vi "Retriggerable_Finite_Counter_20230323_v2019.vi"() -> ()   [LabVIEW 2019]
uses:
  <resource>/objmgr/daqmx.rc
  <vilib>/Utility/error.llb/DialogType.ctl
  <vilib>/DAQmx/configure/timing.llb/DAQmx Timing (Sample Clock).vi
  <vilib>/DAQmx/create/channels.llb/DAQmx Create Channel (CI-Count Edges).vi
  <vilib>/DAQmx/read.llb/DAQmx Read (Counter 1D U32 1Chan NSamp).vi
  <vilib>/DAQmx/create/channels.llb/DAQmx Create Channel (AI-Voltage-Basic).vi
  <vilib>/DAQmx/configure/timing.llb/DAQmx Timing (Implicit).vi
  <vilib>/DAQmx/create/channels.llb/DAQmx Create Channel (CO-Pulse Generation-Frequency).vi
  <vilib>/DAQmx/read.llb/DAQmx Read (Analog 1D Wfm NChan NSamp).vi
  <vilib>/DAQmx/configure/events/hardwareSignals.llb/DAQmx Export Signal (Most Signals).vi
panel:
  in  "AI Physical Channel":tag="Dev2/ai0"
  out "Read Iteration.":i32=20 caption="Read Iteration.\nIf working correctly,\nthis should increment\nonce per second."
  out "Actual Duty Cycle":dbl=0.01
  out "Actual Frequency":dbl=1.0
  in  "Duty Cycle":dbl=0.01 caption="Duty Cycle Must Be Less Than Sampling Duration (%)" format="%.6f"
  in  "Frequency (Hz)":dbl=1.0 format="%.6f"
  in  "Output Terminal":tag="/Dev2/PFI12" caption="Output Terminal For Routing to First Counter"
  in  "Counter 2":tag="Dev2/ctr1"
  out "Total Count\nThis is the":u32 caption="Total Count.\nThis is what you're most interested in."
  in  "Stop":bool
  in  "Trigger Type":enum32{"No Trigger", "Digital Arm Start"}(tab)=enum."Digital Arm Start"
  in  "Edge":i32(ring)=10280 items=["Rising"=10280, "Falling"=10171]
  out "Data":u32[](array[numeric])
  in  "Samples":i32=1000
  in  "Signal Input Terminal":tag="PFI8"
  in  "Counter":tag="Dev2/ctr0"
  in  "Sample Rate":dbl=100000.0
  in  "Sample Clock Source":tag="/Dev2/PFI14"
  # "Task 1: Finite Counter Measurement"
  # "Task 2: Create Sample Clock"
  # "Task 2: Create Slow Pulse Train"
  # "Lots of count values. (You can delete this indicator.\nI've left it here to make it easier to understand how this is working.)"
  # "To configure and use a trigger or the count reset you must have the \"Digital Arm Start\"  tab selected."
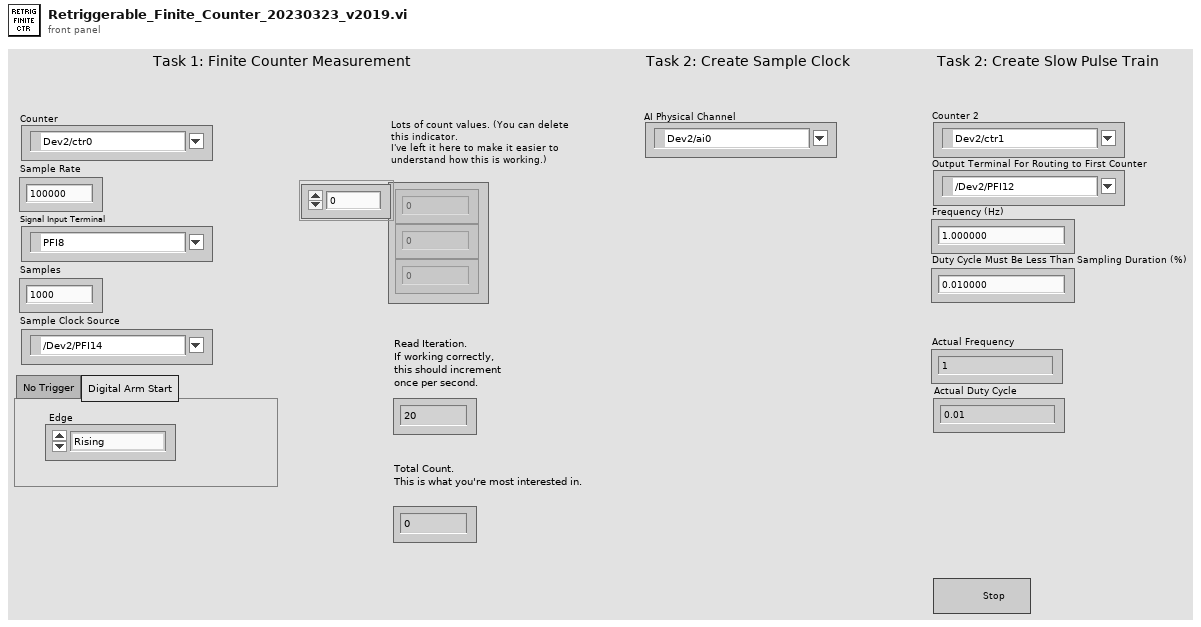
[diagram p1: front panel]
types:
  T1 = typedef "DialogType.ctl" = u16
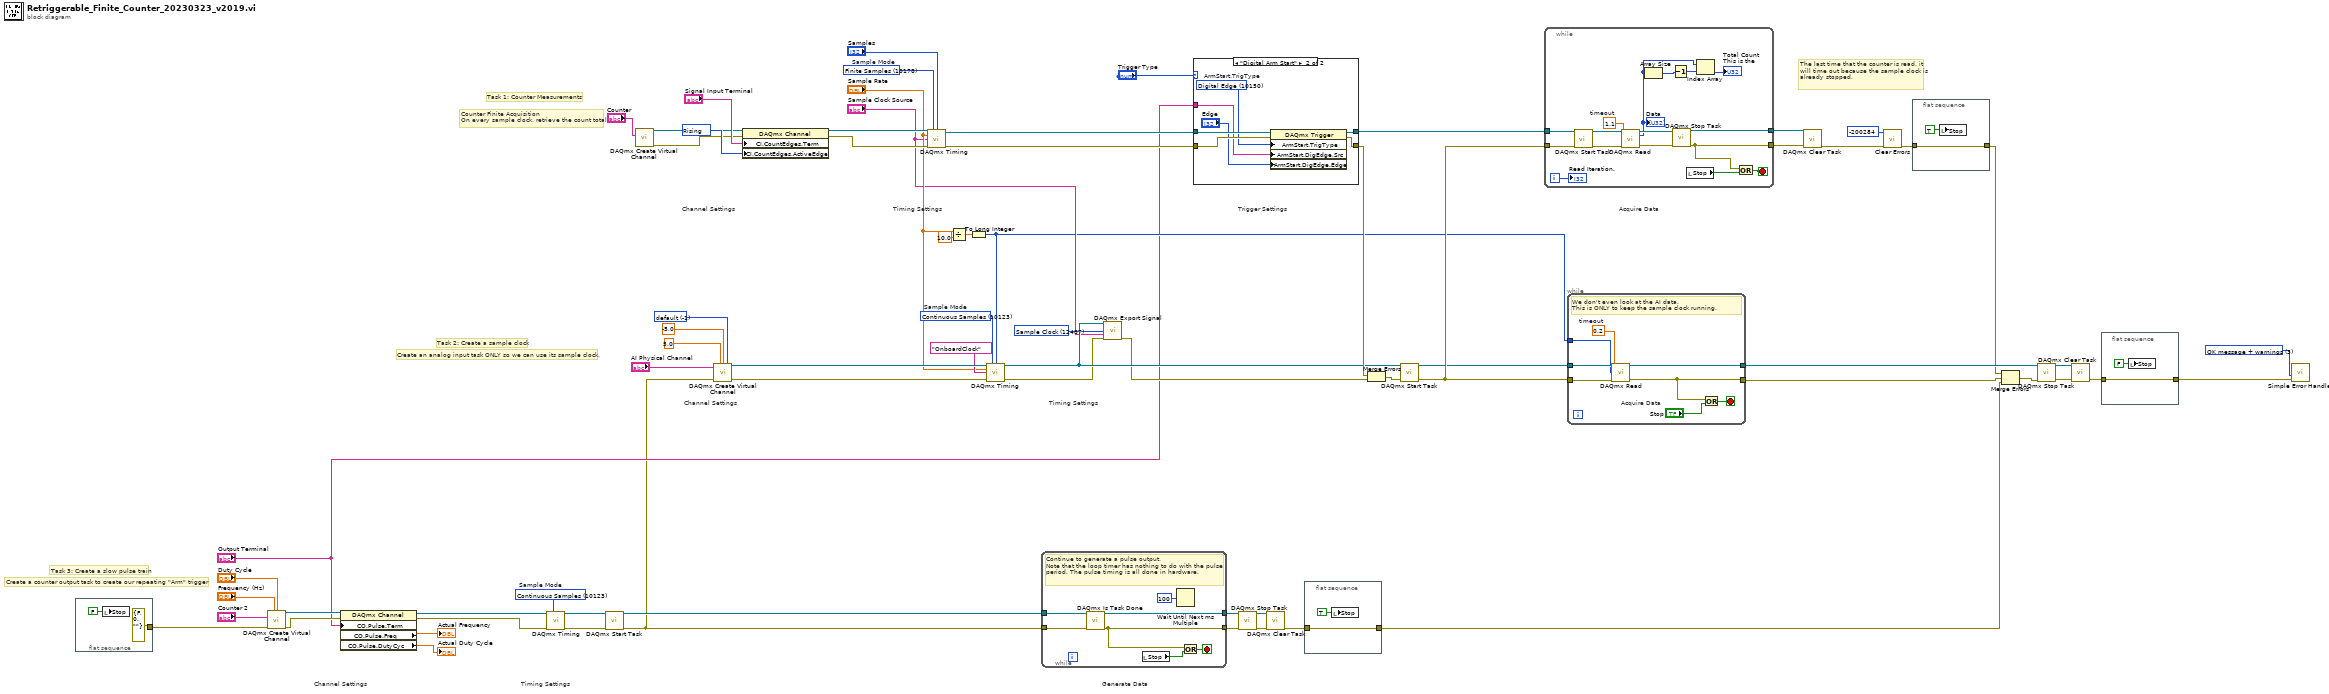
[diagram p0: block diagram]
diagram:
  w69 = 10280 items=["Rising"=10280, "Falling"=10171] ("Active Edge")
  w27 = 10123 items=["Finite Samples"=10178, "Continuous Samples"=10123, "Hardware Timed Single Point"=12522]  # Sample Mode
  w33 = 12487 items=["AI Convert Clock"=12484, "10MHz Reference Clock"=12536, "20MHz Timebase Clock"=12486, "Sample Clock"=12487, "Advance Trigger"=12488, "Reference Trigger"=12490, "Start Trigger"=12491, "Advance Complete Event"=12492, "AI Hold Complete Event"=12493, "Counter Output Event"=12494, "Change Detection Event"=12511, "Watchdog Timer Expired Event"=12512] ("signal")
  w53 = -1 items=["default"=-1, "RSE"=10083, "NRSE"=10078, "Differential"=10106, "Pseudodifferential"=12529] ("Terminal Configuration")
  w46 = T1 3 items=["no dialog", "OK message", "continue or stop message", "OK message + warnings", "continue/stop + warnings"] ("type of dialog (OK msg:1)")
  w57 = 10123 items=["Finite Samples"=10178, "Continuous Samples"=10123, "Hardware Timed Single Point"=12522]  # Sample Mode
  w68 = 10178 items=["Finite Samples"=10178, "Continuous Samples"=10123, "Hardware Timed Single Point"=12522]  # Sample Mode
  # "Task 3: Create a slow pulse train"
  # "Task 2: Create a sample clock"
  # "Task 1: Counter Measurements"
  # "The last time that the counter is read, it will time out because the sample clock is already stopped."
  # "Create a counter output task to create our repeating \"Arm\" trigger"
  # "Generate Data"
  # "Timing Settings"
  # "Channel Settings"
  # "Create an analog input task ONLY so we can use its sample clock."
  # "Counter Finite Acquisition\nOn every sample clock, retrieve the count total"
  # "Acquire Data"
  # "Timing Settings"
  # "Channel Settings"
  # "Acquire Data"
  # "Trigger Settings"
  # "Timing Settings"
  # "Channel Settings"
  n1 = flat-sequence {
    tunnel: [errorcluster {"status"=FALSE, "code"=0, "source"=""} ("error out")] -> w6
    frame #0 {
      n2 = local write "Stop"(FALSE ("Stop")) -> ()
    }
  }
  n3 = call-poly <vilib>:"DAQmx Create Virtual Channel.vi"("frequency"="Frequency (Hz)", "duty cycle"="Duty Cycle", "counter"="Counter 2", "error in"=w6) -> ("task out"=w22:refnum<k21>, "error out"=w21:errorcluster)  [unwired: 10 in]
  n4 = property class="DAQmx Channel"(reference=w22, error in=w21, "CO.Pulse.Term"="Output Terminal") -> (reference out=w19:refnum<k21>, error out=w20:errorcluster, "CO.Pulse.Freq"=→"Actual Frequency":dbl, "CO.Pulse.DutyCyc"=→"Actual Duty Cycle":dbl)
  n5 = call-poly <vilib>:"DAQmx Timing.vi"("task/channels in"=w19, "sample mode"=w27, "error in"=w20) -> ("task out"=w24:refnum<k21>, "error out"=w23:errorcluster)  [unwired: 11 in]
  n6 = call <vilib>:"DAQmx Start Task.vi"("task/channels in"=w24, "error in"=w23) -> ("task out"=w26:refnum<k21>, "error out"=w7:errorcluster)  [unwired: 12 in]
  n7 = call-poly <vilib>:"DAQmx Create Virtual Channel.vi"("counter"="Counter") -> ("task out"=w66:refnum<k21>, "error out"=w63:errorcluster)  [unwired: 13 in]
  n8 = call-poly <vilib>:"DAQmx Create Virtual Channel.vi"("maximum value"=5.0 ("Max Voltage"), "minimum value"=-5.0 ("Min Voltage"), "input terminal configuration"=w53, "physical channels"="AI Physical Channel", "error in"=w7) -> ("task out"=w55:refnum<k21>, "error out"=w56:errorcluster)  [unwired: 9 in]
  n9 = property class="DAQmx Channel"(reference=w66, error in=w63, "CI.CountEdges.Term"="Signal Input Terminal", "CI.CountEdges.ActiveEdge"=w69) -> (reference out=w65:refnum<k21>, error out=w64:errorcluster)
  n10 = call-poly <vilib>:"DAQmx Timing.vi"("task/channels in"=w65, "sample mode"=w68, "samples per channel"="Samples", "rate"="Sample Rate", "source"="Sample Clock Source", "error in"=w64) -> ("task out"=w59:refnum<k21>, "error out"=w60:errorcluster)  [unwired: 8 in]
  n11 = Divide(x="Sample Rate", y=10.0) -> (x/y=w37:dbl)
  n12 = To Long Integer(number=w37) -> (32bit integer=w30:i32)
  n13 = call-poly <vilib>:"DAQmx Timing.vi"("task/channels in"=w55, "sample mode"=w57, "samples per channel"=w30, "rate"="Sample Rate", "source"=tag "OnboardClock" ("Sample Clock Source 2"), "error in"=w56) -> ("task out"=w36:refnum<k21>, "error out"=w35:errorcluster)  [unwired: 8 in]
  n14 = while {
    tunnel: w26 -> [w79]
    tunnel: w7 -> [w78]
    tunnel: [w75] -> w11
    tunnel: [w76] -> w12
    stop <- w77 stop-if-true
    # "Continue to generate a pulse output. \nNote that the loop timer has nothing to do with the pulse period. The pulse timing is all done in hardware."
    n15 = call <vilib>:"DAQmx Is Task Done.vi"("task/channels in"=w79, "error in"=w78) -> ("task out"=w76:refnum<k21>, "error out"=w75:errorcluster)  [unwired: 11 in, 1 out]
    n16 = local read "Stop"() -> (w73:bool)
    n17 = Wait Until Next ms Multiple(millisecond multiple=u32 100) -> ()  [unwired: 1 out]
    n18 = Or(x=w75, y=w73) -> (x .or. y?=w77:bool)
  }
  n19 = call-poly <vilib>:"DAQmx Export Signal.vi"("task/channels in"=w36, "signal"=w33, "output terminal"="Sample Clock Source", "error in"=w35) -> ("error out"=w34:errorcluster)  [unwired: 10 in, 1 out]
  n20 = case shown="\"Digital Arm Start\"" "Trigger Type" {
    tunnel: w59 -> [w81 w88]
    tunnel: w60 -> [w80 w85]
    tunnel: [w81 w87] -> w58
    tunnel: [w80 w86] -> w44
    tunnel: "Output Terminal" -> [_ w82]
    frame "No Trigger", Default {
    }
    frame "Digital Arm Start" {
      w83 = 10150 items=["Digital Edge"=10150, "None"=10230]  # ArmStart.TrigType
      n21 = property class="DAQmx Trigger"(reference=w88, error in=w85, "ArmStart.TrigType"=w83, "ArmStart.DigEdge.Src"=w82, "ArmStart.DigEdge.Edge"="Edge") -> (reference out=w87:refnum<k21>, error out=w86:errorcluster)
    }
  }
  n22 = call <vilib>:"DAQmx Stop Task.vi"("task/channels in"=w12, "error in"=w11) -> ("task out"=w14:refnum<k21>, "error out"=w13:errorcluster)  [unwired: 12 in]
  n23 = call <vilib>:"DAQmx Clear Task.vi"("task in"=w14, "error in"=w13) -> ("error out"=w9:errorcluster)  [unwired: 13 in]
  n24 = flat-sequence {
    tunnel: [w89] -> w8
    tunnel: w9 -> [w89]
    frame #0 {
      n25 = local write "Stop"(TRUE ("Stop")) -> ()
    }
  }
  n26 = Merge Errors(w44, w34) -> (w45:errorcluster)
  n27 = call <vilib>:"DAQmx Start Task.vi"("task/channels in"=w36, "error in"=w45) -> ("task out"=w31:refnum<k21>, "error out"=w43:errorcluster)  [unwired: 12 in]
  n28 = while {
    tunnel: w58 -> [w104]
    tunnel: [w93] -> w5
    tunnel: [w92] -> w4
    tunnel: w43 -> [w101]
    i -> [w94]
    stop <- w96 stop-if-true
    w91 = 1.1  # timeout
    n29 = call <vilib>:"DAQmx Start Task.vi"("task/channels in"=w104, "error in"=w101) -> ("task out"=w106:refnum<k21>, "error out"=w105:errorcluster)  [unwired: 12 in]
    n30 = call-poly <vilib>:"DAQmx Read.vi"("task/channels in"=w106, "timeout"=w91, "error in"=w105) -> ("task out"=w102:refnum<k21>, "data"=w98:u32[], "error out"=w103:errorcluster)  [unwired: 10 in]
    "Data" <- w98
    n31 = Array Size(array=w98) -> (size(s)=w100:i32)
    n32 = Decrement(x=w100) -> (x-1=w99:i32)
    n33 = call <vilib>:"DAQmx Stop Task.vi"("task/channels in"=w102, "error in"=w103) -> ("task out"=w93:refnum<k21>, "error out"=w92:errorcluster)  [unwired: 12 in]
    n34 = local read "Stop"() -> (w95:bool)
    n35 = Index Array(array=w98, index=w99) -> (element=→"Total Count\nThis is the":u32)
    n36 = Or(x=w92, y=w95) -> (x .or. y?=w96:bool)
    "Read Iteration." <- w94
  }
  n37 = while {
    tunnel: w31 -> [w114]
    tunnel: w43 -> [w113]
    tunnel: [w112] -> w49
    tunnel: [w110] -> w42
    tunnel: w30 -> [w108]
    stop <- w109 stop-if-true
    w107 = 0.2  # timeout
    # "We don't even look at the AI data.\nThis is ONLY to keep the sample clock running."
    n38 = call-poly <vilib>:"DAQmx Read.vi"("task/channels in"=w114, "number of samples per channel"=w108, "timeout"=w107, "error in"=w113) -> ("task out"=w112:refnum<k21>, "error out"=w110:errorcluster)  [unwired: 9 in, 1 out]
    n39 = Or(x=w110, y="Stop") -> (x .or. y?=w109:bool)
  }
  n40 = call <vilib>:"DAQmx Clear Task.vi"("task in"=w5, "error in"=w4) -> ("error out"=w3:errorcluster)  [unwired: 13 in]
  n41 = call <vilib>:"Clear Errors.vi"("error in (no error)"=w3, "specific error code to clear (0: all)"=-200284) -> ("error out"=w2:errorcluster)  [unwired: 4 in, 1 out]
  n42 = flat-sequence {
    tunnel: [w115] -> w40
    tunnel: w2 -> [w115]
    frame #0 {
      n43 = local write "Stop"(TRUE ("Stop")) -> ()
    }
  }
  n44 = Merge Errors(w40, w42, w8) -> (w41:errorcluster)
  n45 = call <vilib>:"DAQmx Stop Task.vi"("task/channels in"=w49, "error in"=w41) -> ("task out"=w47:refnum<k21>, "error out"=w48:errorcluster)  [unwired: 12 in]
  n46 = call <vilib>:"DAQmx Clear Task.vi"("task in"=w47, "error in"=w48) -> ("error out"=w29:errorcluster)  [unwired: 13 in]
  n47 = flat-sequence {
    tunnel: [w117] -> w28
    tunnel: w29 -> [w117]
    frame #0 {
      n48 = local write "Stop"(FALSE ("Stop")) -> ()
    }
  }
  n49 = call <vilib>:"Simple Error Handler.vi"("type of dialog (OK msg:1)"=w46, "error in (no error)"=w28) -> ()  [unwired: 3 in, 5 out]
